vi "Signal Analyzer2.vi"() -> ()   [LabVIEW 2014]
panel:
  out "Waveform Graph":dynamicdata(graph)
  out "Phase 2":dbl
  out "Frequency 3":dbl
  out "Amplitude 2":dbl
  out "Phase":dbl
  out "Frequency 2":dbl
  out "Amplitude":dbl
  in  "Frequency":dbl=1.0
  in  "stop":bool
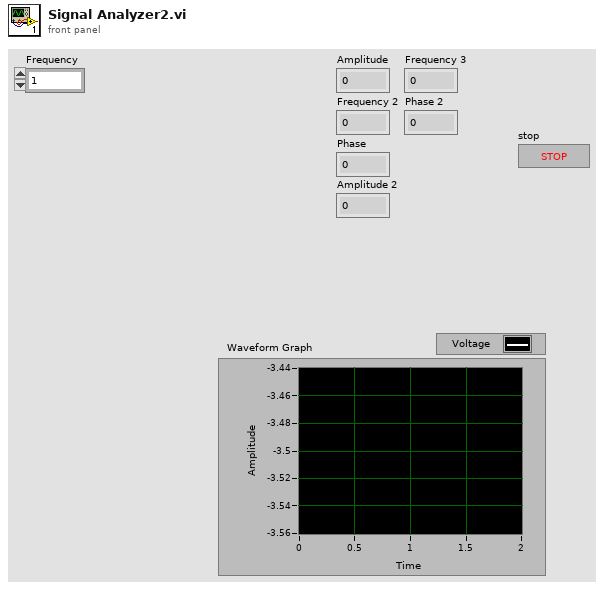
[diagram p1: front panel]
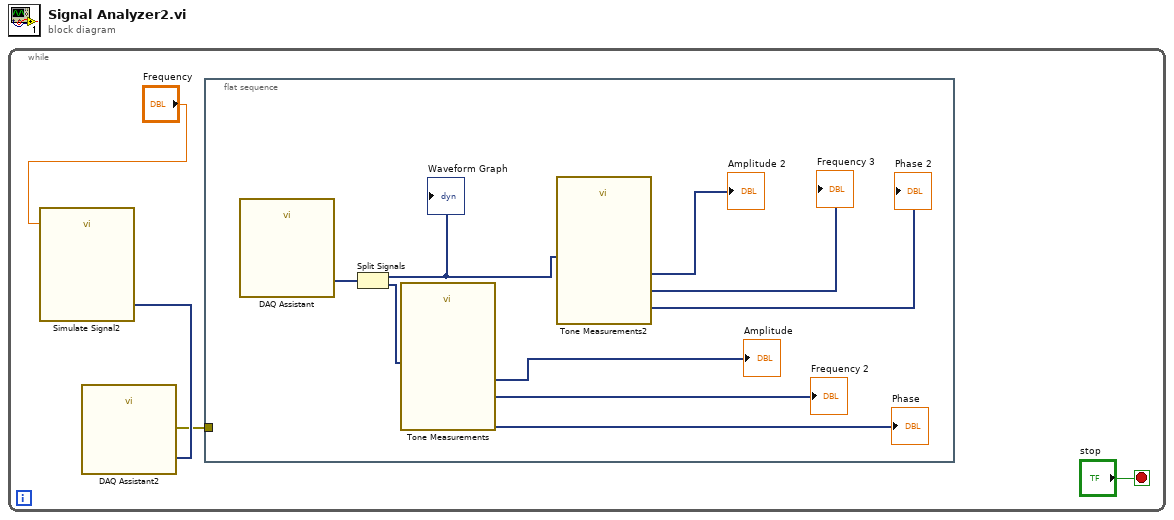
[diagram p0: block diagram]
diagram:
  n1 = while {
    stop <- "stop" stop-if-true
    n2 = call "Simulate Signal2"("Frequency"="Frequency") -> ("Sine"=w3:dynamicdata)  [unwired: 13 in, 1 out]
    n3 = call "DAQ Assistant2"("data"=w3) -> ("error out"=w1:errorcluster)  [unwired: 16 in, 2 out]
    n4 = flat-sequence {
      tunnel: w1 -> [_]
      frame #0 {
        n5 = call "DAQ Assistant"() -> ("data"=w13:dynamicdata)  [unwired: 16 in, 3 out]
        n6 = Split Signals(w13) -> (w11:dynamicdata, w12:dynamicdata)  [unwired: 2 in]
        "Waveform Graph" <- w11
        n7 = call "Tone Measurements"("Signals"=w12) -> ("Phase"=→"Phase":dynamicdata, "Frequency"=→"Frequency 2":dynamicdata, "Amplitude"=→"Amplitude":dynamicdata)  [unwired: 7 in, 1 out]
        n8 = call "Tone Measurements2"("Signals"=w11) -> ("Phase"=→"Phase 2":dynamicdata, "Frequency"=→"Frequency 3":dynamicdata, "Amplitude"=→"Amplitude 2":dynamicdata)  [unwired: 7 in, 1 out]
      }
    }
  }
